vi "Storage Vacuum Global.vi"(7 "Action":enum16{"Initialize", "Read", "Write"}(ring)=enum."Write", 8 "error in (no error)":errorcluster, 10 "Write":bool=TRUE, 11 "Carrier Tray.lvclass":refnum<class "Assembly Tray.lvclass">) -> (0 "error out":errorcluster, 2 "Read":bool, 3 "Carrier Tray.lvclass 2":refnum<class "Assembly Tray.lvclass">)   [LabVIEW 2020, in "Assembly Tray.lvclass"]
uses:
  Assembly Tray.lvclass
  C:/Users/hep/Documents/CMU gantry/Classes/Workspace/Fixture.lvclass
  Fixture.lvclass/Fixture.ctl
  Read Fixture ID.vi
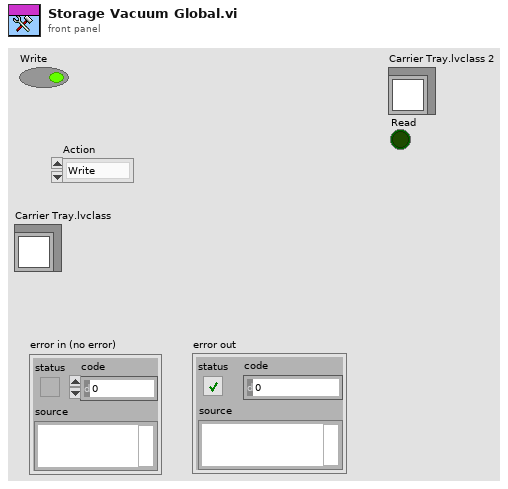
[diagram p1: front panel]
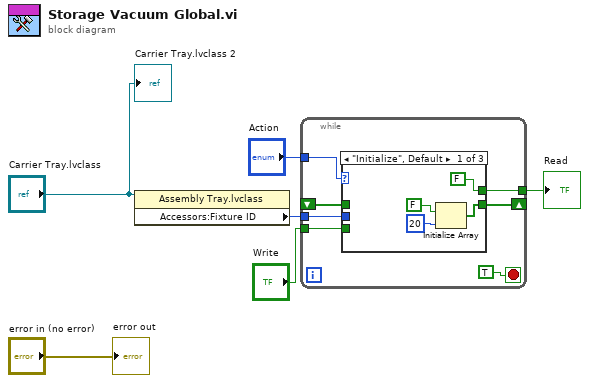
[diagram p0: block diagram]
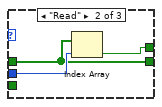
[diagram p2: hidden frame]
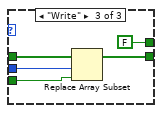
[diagram p3: hidden frame]
diagram:
  n1 = property class="Assembly Tray.lvclass"(reference="Carrier Tray.lvclass") -> ("Accessors:Fixture ID"=w4:i32)  [unwired: 1 in, 2 out]
  n2 = while {
    tunnel: "Action" -> [w12]
    shift-right: [w11] -> _
    shift-left: _ -> [w10]
    tunnel: w4 -> [w9]
    tunnel: [w8] -> w1
    tunnel: "Write" -> [w7]
    stop <- TRUE stop-if-true
    n3 = case shown="\"Initialize\", Default" w12 {
      tunnel: [w14 w18 w22] -> w11
      tunnel: w10 -> [_ w18 w25]
      tunnel: w9 -> [_ w20 w24]
      tunnel: [FALSE w19 FALSE] -> w8
      tunnel: w7 -> [_ _ w23]
      frame "Initialize", Default {
        n4 = Initialize Array(FALSE, 20 ("dimension size")) -> (w14:bool[])
      }
      frame "Read" {
        n5 = Index Array(array=w18, index=w20) -> (element=w19:bool)
      }
      frame "Write" {
        n6 = Replace Array Subset(array=w25, new element=w23, index=w24) -> (w22:bool[])
      }
    }
  }
  "Read" <- w1
  "error out" <- "error in (no error)"
  "Carrier Tray.lvclass 2" <- "Carrier Tray.lvclass"
